vi "Test.vi"() -> ()   [LabVIEW 2020, in "EPA 1065.lvlib" / "T90 Test 1065-308.lvlib"]
uses:
  T90 Test 1065-308.lvlib
  T90 Konfig Daten.ctl
  Modus.ctl
  Seiten/System Einstellungen V2/Analysatoren.ctl
  Seiten/System Einstellungen V2/Gasflasche Auswahl.ctl
  Seiten/System Einstellungen V2/Konfig Gasflasche.ctl
  Frequenz.ctl
  Seiten/System Einstellungen V2/System Einstellungen V2.lvlib
panel:
  out "Tabellen-String":string
  out "Array":string[](array[string])
  in  "T90 Konfig Daten":T1={"Bearbeiter:"="", "Komponente:"=0, "Gasflaschen Nr.:"="", "Accuracy"=0.0, "Sollwert"=0.0, "Modus"=0, "Abschaltzeit:"=120.0, "Abweichung:"=3.0, "Pfad:"=path "D:/IAG_Data/Log", "Textname:"="", "CG Aufschaltzeit:"=120.0, "Einheit"="", "N2 Aufschaltzeit:"=120.0, "Analysator"="", "Gasflasche"=0, "Konfig Gasflasche"=FALSE, "Frequency:"=5} {"Frequency:" items=["5 Hz"=5, "10 Hz"=10]; "Gasflasche" items=["----"=10000, "IAG NH3 3000"=0, "IAG NH3 200"=1, "IAG NH3 2000"=2, "IAG MG"=3, "IAG O2"=4]; "N2 Aufschaltzeit:" min=60.0; "CG Aufschaltzeit:" min=60.0; "Abweichung:" min=2.0; "Abschaltzeit:" min=60.0; "Modus" items=["CG zu PNS", "CG zu Entnahmestelle"]}
  in  "Stopp":bool
  in  "Boolesch":bool
  out "TestStatus":string
  # "sec."
  # "sec."
  # "%"
  # "%"
  # "sec."
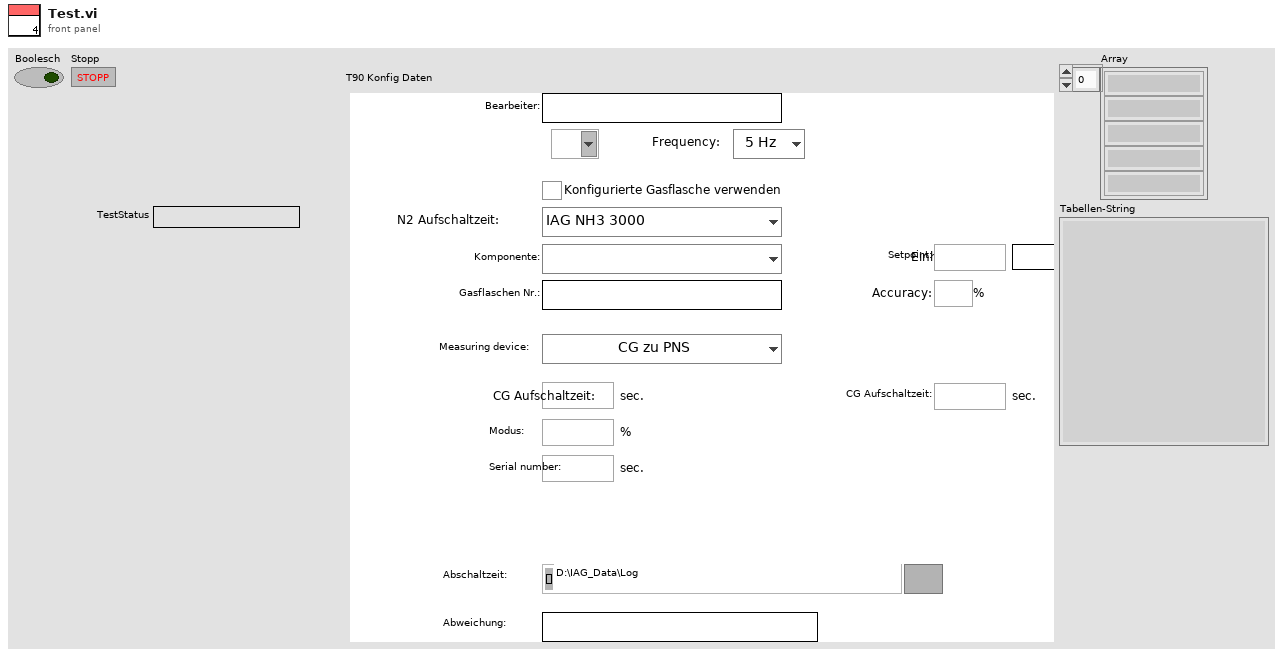
[diagram p1: front panel]
types:
  T1 = typedef "EPA 1065.lvlib/T90 Test 1065-308.lvlib/T90 Konfig Daten.ctl" = cluster{"Bearbeiter:":string, "Komponente:":u16, "Gasflaschen Nr.:":string, "Accuracy":dbl, "Sollwert":dbl, "Modus":T2, "Abschaltzeit:":dbl, "Abweichung:":dbl, "Pfad:":path, "Textname:":string, "CG Aufschaltzeit:":dbl, "Einheit":string, "N2 Aufschaltzeit:":dbl, "Analysator":T3, "Gasflasche":T4, "Konfig Gasflasche":T5, "Frequency:":T6}
  T2 = typedef "EPA 1065.lvlib/T90 Test 1065-308.lvlib/Modus.ctl" = u16
  T3 = typedef "System Einstellungen V2.lvlib/Analysatoren.ctl" = string
  T4 = typedef "System Einstellungen V2.lvlib/Gasflasche Auswahl.ctl" = u16
  T5 = typedef "System Einstellungen V2.lvlib/Konfig Gasflasche.ctl" = bool
  T6 = typedef "EPA 1065.lvlib/T90 Test 1065-308.lvlib/Frequenz.ctl" = u16
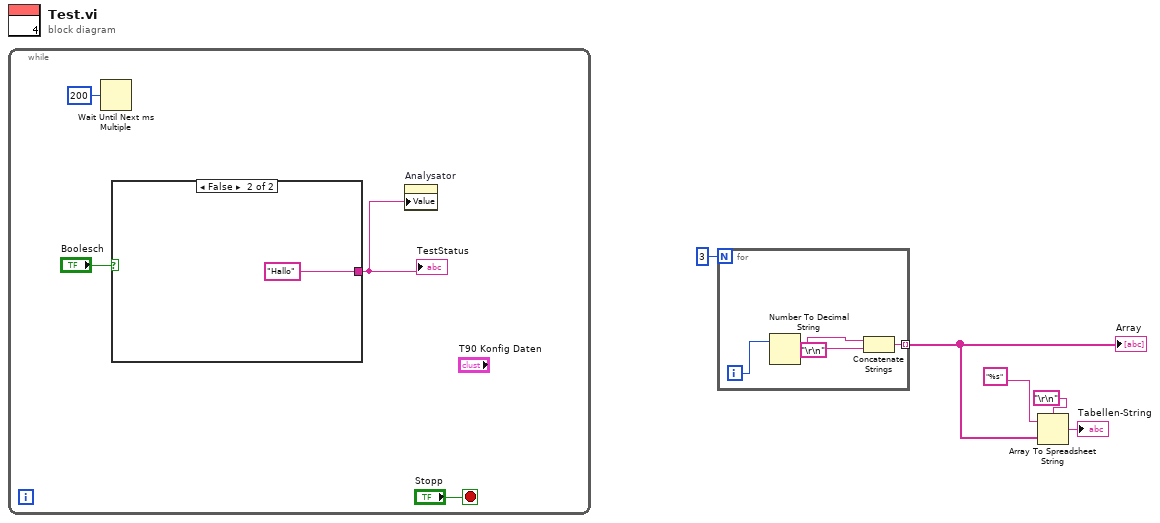
[diagram p0: block diagram]
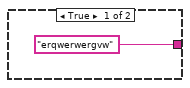
[diagram p2: hidden frame]
diagram:
  n1 = while {
    stop <- "Stopp" stop-if-true
    n2 = Wait Until Next ms Multiple(millisecond multiple=u32 200 ("ms")) -> ()  [unwired: 1 out]
    n3 = case shown="False" "Boolesch" {
      tunnel: ["erqwerwergvw" ("TestStatus") "Hallo" ("TestStatus")] -> w6
      frame True {
      }
      frame False {
      }
    }
    "TestStatus" <- w6
    n4 = property on="Analysator" class="KombiFeld (strikt)"("Value"=w6) -> ()  [unwired: 2 in, 2 out]
  }
  n5 = for {
    N: 3 -> [_]
    tunnel: [w12] -> w2 mode=indexing
    i -> [w15]
    n6 = Number To Decimal String(number=w15) -> (decimal integer string=w13:string)  [unwired: 1 in]
    n7 = Concatenate Strings(w13, "\r\n") -> (w12:string)
  }
  "Array" <- w2
  n8 = Array To Spreadsheet String(delimiter (Tab)="\r\n", array=w2, 3:"%s" ("Format-String")) -> (spreadsheet string=→"Tabellen-String":string)
